vi "Find Zombies.vi"(8 "Error In":errorcluster, 11 "VI In":refnum<vi>) -> (0 "Error Out":errorcluster, 2 "Zombies":refnum<vi>[](array[refnum]), 3 "VI Out":refnum<vi>)   [LabVIEW 2017, in "Toolkit.lvlib"]
doc: "Finds all zombies in the block diagram of a VI."
uses:
  Toolkit.lvlib
  <vilib>/Utility/traverseref.llb/TRef TravTarget.ctl
  <vilib>/Utility/traverseref.llb/VI Scripting - Traverse.lvlib
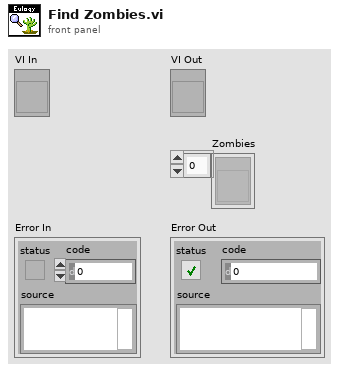
[diagram p1: front panel]
types:
  T1 = typedef "TRef TravTarget.ctl" = enum16{"FP", "BD", "Other"}
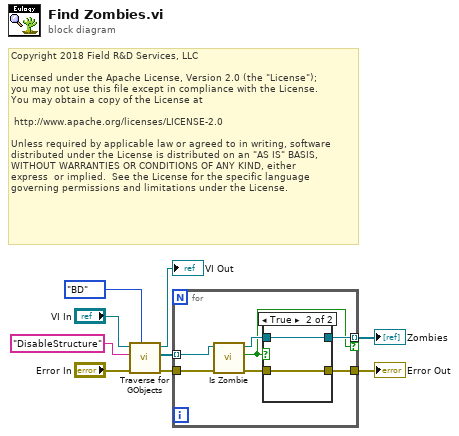
[diagram p0: block diagram]
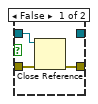
[diagram p2: hidden frame]
diagram:
  # "Copyright 2018 Field R&D Services, LLC\n\nLicensed under the Apache License, Version 2.0 (the \"License\");\nyou may not use this file except in compliance with the License.\nYou may obtain a copy of the License at\n\n\thttp://www.apache.org/licenses/LICENSE-2.0\n\nUnless required by applicable law or agreed to in writing, software\ndistributed under the License is distributed on an \"AS IS\" BASIS,\nWITHOUT WARRANTIES OR CONDITIONS OF ANY KIND, either \nexpress  or implied.  See the License for the specific language \ngoverning permissions and limitations under the License."
  n1 = call <vilib>:"Traverse for GObjects.vi"("Traverse Target"=TRef_TravTarget."BD", "error in (no error)"="Error In", "Class Name"="DisableStructure", "VI Refnum"="VI In") -> ("error out"=w5:errorcluster, "References"=w4:refnum<vi>[], "dup VI Refnum"=→"VI Out":refnum<vi>)  [unwired: 4 in, 1 out]
  n2 = for {
    tunnel: w5 -> [w16]
    tunnel: w4 -> [w15] mode=indexing
    tunnel: [w13] -> w3 mode=indexing if=w12
    tunnel: [w10] -> w2
    n3 = call "Is Zombie.vi"("Error In"=w16, "GObject In"=w15) -> ("Error Out"=w11:errorcluster, "Zombie?"=w12:bool, "GObject Out"=w14:refnum<vi>)  [unwired: 7 in]
    n4 = case shown="True" w12 {
      tunnel: w14 -> [w19 w21]
      tunnel: [_ w21] -> w13
      tunnel: w11 -> [w18 w20]
      tunnel: [w17 w20] -> w10
      frame False {
        n5 = Close Reference(reference=w19, error in (no error)=w18) -> (error out=w17:errorcluster)
      }
      frame True {
      }
    }
  }
  "Zombies" <- w3
  "Error Out" <- w2
